vi "AVS_Deactivate.vi"(0 "a_hHandle":i32) -> (4 "Output Value":i32)   [LabVIEW 2013, in "Avantes Spectrometer Functions.lvlib"]
uses:
  Avantes Spectrometer Functions.lvlib
  AS5216.dll
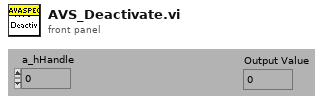
[diagram p1: front panel]
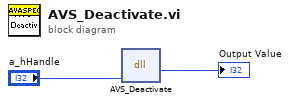
[diagram p0: block diagram]
diagram:
  n1 = dll-call lib="C:/Users/dhstuart/Dropbox/CLTC/avantesSpectrometer/Libraries/polling_mc/AS5216.dll" fn="AVS_Deactivate"("a_hHandle"="a_hHandle") -> (→"Output Value":i32)  [unwired: 4 in, 2 out]
